vi "5 Ball Limit global.vi"() -> ()   [LabVIEW 2019]
panel:
  in  "5 Ball Limit":bool
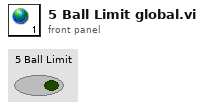
[diagram p1: front panel]
diagram:
